vi "RC_test_reader.vi"(8 "error in (no error)":errorcluster, 9 "Motors IDs Found":u8[](array[numeric]), 10 "Read positions (dyn)":dbl[](array[numeric]), 11 "VISA Refnum in":refnum<visa-resource-name>) -> (0 "error out":errorcluster[](array[cluster]), 1 "Motors Read Correctly":bool[](array[boolean]), 2 "Dynamixel Positions (deg)":dbl[](array[numeric]), 3 "Read positions latest (dyn)":dbl[](array[numeric]), 5 "VISA Refnum OUT":refnum<visa-resource-name>)   [LabVIEW 2013]
doc: "This VI takes an array of motor IDs and reads the position of each one. It outputs as both raw values and as degrees.\n\nIt's set up for the SAIL Dynamixels, because it scales by 360/1200. We're still investigating whether the rudder has different units."
uses:
  <instrlib>/Dynamixel Motor/Dynamixel Motor.lvlib
panel:
  in  "Rudder ID":u8
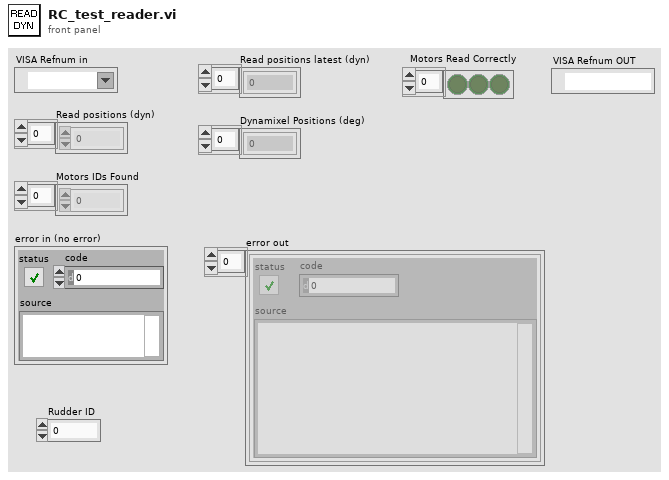
[diagram p1: front panel]
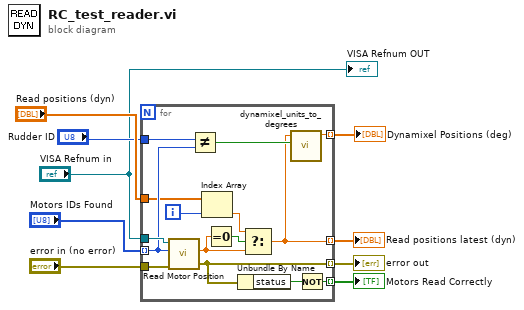
[diagram p0: block diagram]
diagram:
  n1 = for {
    tunnel: "VISA Refnum in" -> [w24]
    tunnel: "Motors IDs Found" -> [w20] mode=indexing
    tunnel: "error in (no error)" -> [w23]
    tunnel: [w15] -> w8 mode=indexing
    tunnel: "Read positions (dyn)" -> [w11]
    tunnel: [w18] -> w5 mode=indexing
    tunnel: [w17] -> w4 mode=indexing
    tunnel: "Rudder ID" -> [w16]
    tunnel: [w13] -> w2 mode=indexing
    i -> [w12]
    n2 = call <instrlib>:"Read Motor Position.vi"("error in (no error)"=w23, "Motor ID (0)"=w20, "VISA resource name"=w24) -> ("error out"=w15:errorcluster, "Position (deg)"=w21:dbl)  [unwired: 6 in, 1 out]
    n3 = Not Equal?(x=w16, y=w20) -> (x != y?=w19:bool)
    n4 = Index Array(array=w11, index=w12) -> (element=w10:dbl)
    n5 = Equal To 0?(x=w21) -> (x = 0?=w22:bool)
    n6 = Unbundle By Name(w15) -> ("status"=w14:bool)
    n7 = Select(t=w10, s=w22, f=w21) -> (s? t:f=w18:dbl)
    n8 = call "dynamixel_units_to_degrees.vi"("MX Motor? (T)"=w19, "Dynamixel Input"=w18) -> ("Degrees"=w17:dbl)  [unwired: 8 in, 1 out]
    n9 = Not(x=w14) -> (.not. x?=w13:bool)
  }
  "Read positions latest (dyn)" <- w5
  "Dynamixel Positions (deg)" <- w4
  "error out" <- w8
  "Motors Read Correctly" <- w2
  "VISA Refnum OUT" <- "VISA Refnum in"
